vi "http delete.vi"(0 "url":string, 5 "headers_json":string, 7 "timeout_ms":i32, 11 "error in (no error)":errorcluster) -> (3 "response_len_out out":i32, 4 "function return":i32, 10 "handle_out out":u64, 14 "status_out out":u32, 15 "error out":errorcluster)   [LabVIEW 2020, in "reqwest-labview.lvlib"]
doc: "int http_delete(const char *url,\n const char *headers_json,\n int timeout_ms,\n void **handle_out,\n int *response_len_out,\n unsigned int *status_out);"
uses:
  reqwest-labview.lvlib
  reqwest_labview_64.dll
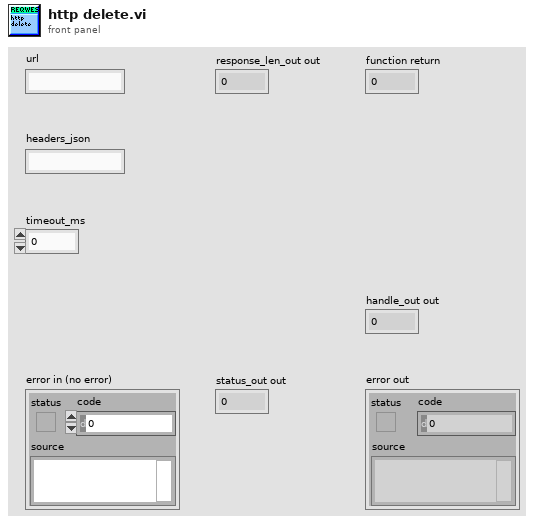
[diagram p1: front panel]
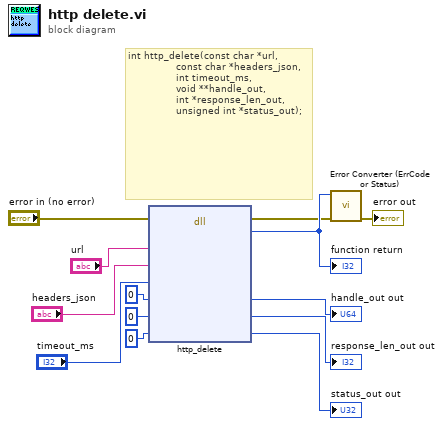
[diagram p0: block diagram]
diagram:
  # "int http_delete(const char *url,\n                const char *headers_json,\n                int timeout_ms,\n                void **handle_out,\n                int *response_len_out,\n                unsigned int *status_out);"
  n1 = dll-call lib="C:/code/reqwest-labview/lv-src/shared-library/reqwest_labview_*.*" fn="http_delete"(error in="error in (no error)", "url"="url", "headers_json"="headers_json", "timeout_ms"="timeout_ms", "handle_out"=u64 0, "response_len_out"=0, "status_out"=u32 0) -> (error out=w2:errorcluster, "return type"=w13:i32, "handle_out"=→"handle_out out":u64, "response_len_out"=→"response_len_out out":i32, "status_out"=→"status_out out":u32)  [unwired: 5 in, 1 out]
  "function return" <- w13
  n2 = call "Error Converter (ErrCode or Status).vi"("error in (no error)"=w2, "error code"=w13) -> ("error out"=→"error out":errorcluster)  [unwired: 9 in]
